vi "stopImaging.vi"(8 "error in (no error)":errorcluster, 11 "Model in":refnum<class "Model.lvclass">) -> (0 "error out":errorcluster, 3 "Model out":refnum<class "Model.lvclass">)   [LabVIEW 2016, in "Model.lvclass"]
uses:
  Model.lvclass
  Model.lvclass/Model.ctl
  ss_sedspectrometer/SEDSpectrometer/FiberSpectrograph.lvclass
  CFitsIO/CFitsIO.lvclass
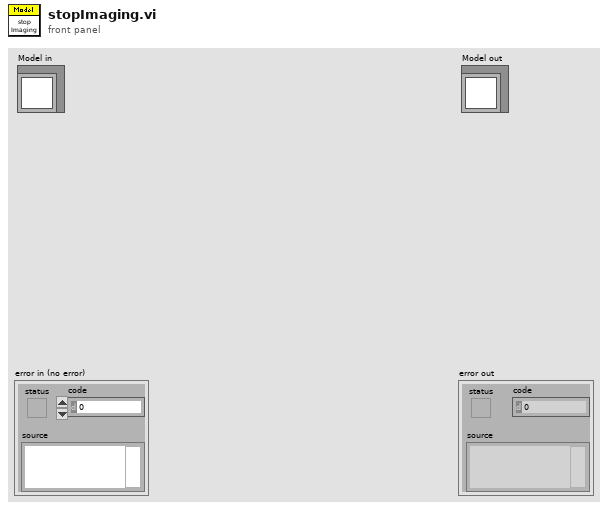
[diagram p1: front panel]
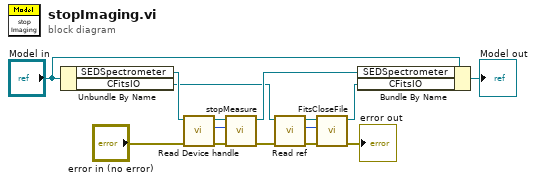
[diagram p0: block diagram]
diagram:
  n1 = Unbundle By Name("Model in") -> ("SEDSpectrometer"=w15:refnum<class "FiberSpectrograph.lvclass">, "CFitsIO"=w6:refnum<class "CFitsIO.lvclass">)
  n2 = call-dynamic "Read Device handle.vi"("error in (no error)"="error in (no error)", "SEDSpectrometer in"=w15) -> ("error out"=w11:errorcluster, "Device handle"=w13:i32, "SEDSpectrometer out"=w14:refnum<class "FiberSpectrograph.lvclass">)  [unwired: 7 in]
  n3 = call "stopMeasure.vi"("error in (no error)"=w11, "Device"=w13, "SEDSpectrometer in"=w14) -> ("error out"=w7:errorcluster, "SEDSpectrometer out"=w10:refnum<class "FiberSpectrograph.lvclass">)  [unwired: 6 in, 1 out]
  n4 = call-dynamic "Read ref .vi"("error in (no error)"=w7, "CFitsIO in"=w6) -> ("error out"=w3:errorcluster, "ref"=w5:u64, "CFitsIO out"=w4:refnum<class "CFitsIO.lvclass">)  [unwired: 7 in]
  n5 = call-dynamic "FitsCloseFile.vi"("error in (no error)"=w3, "ref in"=w5, "CFitsIO in"=w4) -> ("error out"=→"error out":errorcluster, "CFitsIO out"=w1:refnum<class "CFitsIO.lvclass">)  [unwired: 5 in, 2 out]
  n6 = Bundle By Name(cluster="Model in", "SEDSpectrometer"=w10, "CFitsIO"=w1) -> (→"Model out":refnum<class "Model.lvclass">)
